vi "Log.vi"(8 "error in (no error)":errorcluster, 10 "String":string, 11 "Log File Reference":refnum<file>) -> (0 "error out":errorcluster, 3 "Log File Reference":refnum<file>)   [LabVIEW 2011, in "Log VIs.lvlib"]
doc: "Log errors or events to the FOFB Controller log file and console output. The logged information is composed by: timestamp, error code, error description and additional string provided by user (optional)."
uses:
  Log VIs.lvlib
  <vilib>/NI_Real-Time Target Support.lvlib
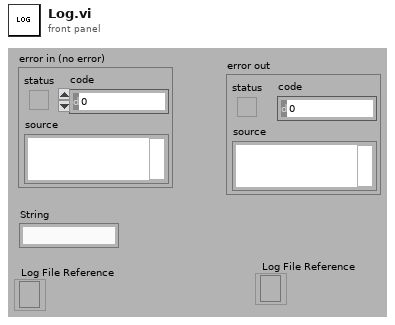
[diagram p1: front panel]
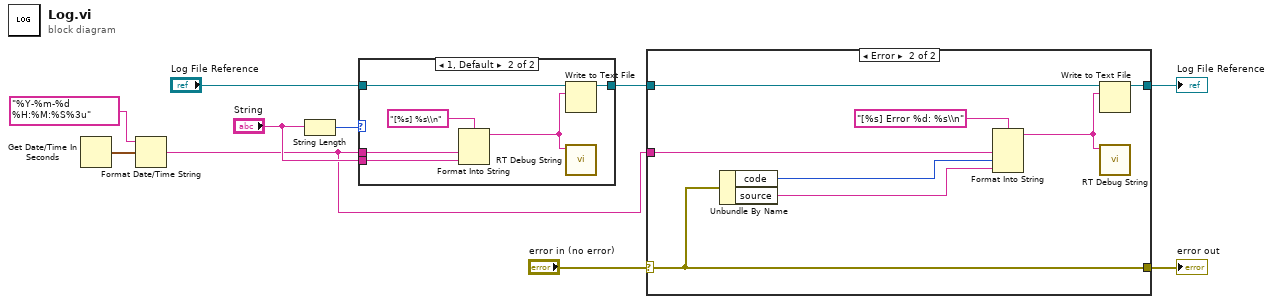
[diagram p0: block diagram]
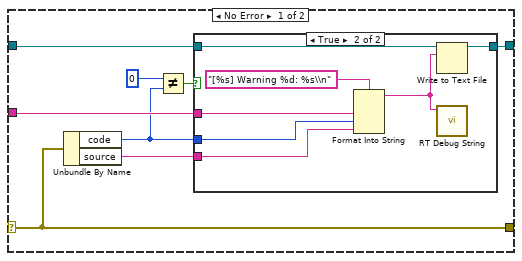
[diagram p3: hidden frame]
diagram:
  n1 = Get Date/Time In Seconds() -> (seconds since 1Jan1904=w7:timestamp)
  n2 = Format Date/Time String(time format string (%c)="%Y-%m-%d %H:%M:%S%3u", seconds (now)=w7) -> (date/time string=w1:string)  [unwired: 1 in]
  n3 = String Length(string="String") -> (length=w5:i32)
  n4 = case shown="1, Default" w5 {
    tunnel: "Log File Reference" -> [w11 w16]
    tunnel: [w11 w15] -> w3
    tunnel: w1 -> [_ w14]
    tunnel: "String" -> [_ w13]
    frame 0 {
    }
    frame 1, Default {
      n5 = Format Into String(format string="[%s] %s\\n" ("initial string"), w14, w13) -> (resulting string=w12:string)  [unwired: 2 in, 1 out]
      n6 = Write to Text File(file (use dialog)=w16, text=w12) -> (refnum out=w15:refnum<file>)  [unwired: 2 in, 2 out]
      n7 = call <vilib>:"RT Debug String.vi"("String to write"=w12) -> ()  [unwired: 10 in, 1 out]
    }
  }
  n8 = case shown="Error" "error in (no error)" {
    selector: "error in (no error)" -> [w23 w39]
    tunnel: [w23 w39] -> w9
    tunnel: w3 -> [w19 w38]
    tunnel: [w18 w37] -> w8
    tunnel: w1 -> [w25 w35]
    frame No Error {
      n9 = Unbundle By Name(w23) -> ("code"=w20:i32, "source"=w24:string)
      n10 = Not Equal?(x=0, y=w20) -> (x != y?=w22:bool)
      n11 = case shown="True" w22 {
        tunnel: w25 -> [_ w31]
        tunnel: w19 -> [w26 w27]
        tunnel: w20 -> [_ w30]
        tunnel: w24 -> [_ w29]
        tunnel: [w26 w28] -> w18
        frame False {
        }
        frame True {
          n12 = Format Into String(format string="[%s] Warning %d: %s\\n" ("initial string"), w31, w30, w29) -> (resulting string=w33:string)  [unwired: 2 in, 1 out]
          n13 = Write to Text File(file (use dialog)=w27, text=w33) -> (refnum out=w28:refnum<file>)  [unwired: 2 in, 2 out]
          n14 = call <vilib>:"RT Debug String.vi"("String to write"=w33) -> ()  [unwired: 10 in, 1 out]
        }
      }
    }
    frame Error {
      n15 = Unbundle By Name(w39) -> ("code"=w41:i32, "source"=w40:string)
      n16 = Format Into String(format string="[%s] Error %d: %s\\n" ("initial string"), w35, w41, w40) -> (resulting string=w34:string)  [unwired: 2 in, 1 out]
      n17 = Write to Text File(file (use dialog)=w38, text=w34) -> (refnum out=w37:refnum<file>)  [unwired: 2 in, 2 out]
      n18 = call <vilib>:"RT Debug String.vi"("String to write"=w34) -> ()  [unwired: 10 in, 1 out]
    }
  }
  "error out" <- w9
  "Log File Reference" <- w8
